vi "Select-Meas. Mode.vi"(7 "clear all channels":bool, 8 "error in (no error)":errorcluster, 9 "comment (\"Setting_1\") (max 58 chars)":string="Setting_1", 10 "measurement mode":bool, 11 "VISA resource name":refnum<visa-resource-name>) -> (0 "error out":errorcluster, 3 "VISA resource name out":refnum<visa-resource-name>)   [LabVIEW 2016, in "Agilent 415X Series.lvlib"]
doc: "This VI selects the measurement mode of the HP415xA."
uses:
  Agilent 415X Series.lvlib
panel:
  # "sampling\nsweep"
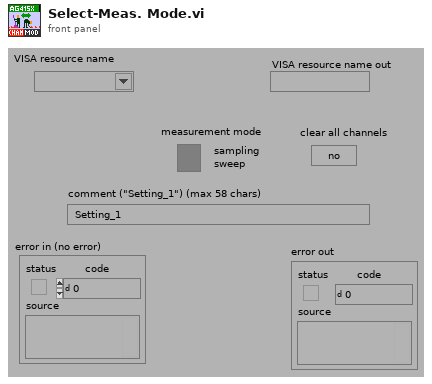
[diagram p1: front panel]
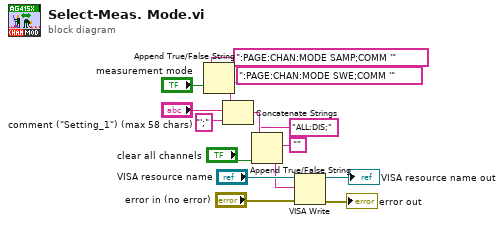
[diagram p0: block diagram]
diagram:
  n1 = Append True/False String(1:"measurement mode", 2:":PAGE:CHAN:MODE SWE;COMM '", 3:":PAGE:CHAN:MODE SAMP;COMM '") -> (0:w8:string)  [unwired: 1 in]
  n2 = Concatenate Strings(w8, "comment (\"Setting_1\") (max 58 chars)", "';") -> (w6:string)
  n3 = Append True/False String(1:"clear all channels", 2:"" ("Empty String Constant"), 3:"ALL:DIS;", 4:w6) -> (0:w5:string)
  n4 = VISA Write(VISA resource name="VISA resource name", write buffer=w5, error in (no error)="error in (no error)") -> (VISA resource name out=→"VISA resource name out":refnum<visa-resource-name>, error out=→"error out":errorcluster)  [unwired: 1 out]
